vi "MGI Append String to Error Source.vi"(4 "Append to Warning? (F)":bool, 6 "Prepend? (F)":bool, 8 "Error In":errorcluster, 9 "String to Append":string) -> (0 "Error Out":errorcluster)   [LabVIEW 2016]
doc: "Append or Prepend the specified message to the input error source string if error exists.\n\nAuthored by Shawn Walpole\nsupport@mooregoodideas.com\nwww.mooregoodideas.com\n\nCopyright (c) 2010, Moore Good Ideas, Inc.\n\nAll rights reserved.\n\nRedistribution and use in source and binary forms, with or without modification, are permitted provided that the following conditions are met:\n\n * Redistributions of source code must retain the above copyright notice, this list of conditions and the following disclaimer.\n * Redistributions in binary form must reproduce the above copyright notice, this list of conditions and the following disclaimer in the documentation and/or other materials provided with the distribution.\n * Neither the name of Moore Good Ideas, Inc. nor the names of its contributors may be used to endorse or promote products derived from this software without specific prior written permission.\n\nTHIS SOFTWARE IS PROVIDED BY THE COPYRIGHT HOLDERS AND CONTRIBUTORS \"AS IS\" AND ANY EXPRESS OR IMPLIED WARRANTIES, INCLUDING, BUT NOT LIMITED TO, THE IMPLIED WARRANTIES OF MERCHANTABILITY AND FITNESS FOR A PARTICULAR PURPOSE ARE DISCLAIMED. IN NO EVENT SHALL THE COPYRIGHT OWNER OR CONTRIBUTORS BE LIABLE FOR ANY DIRECT, INDIRECT, INCIDENTAL, SPECIAL, EXEMPLARY, OR CONSEQUENTIAL DAMAGES (INCLUDING, BUT NOT LIMITED TO, PROCUREMENT OF SUBSTITUTE GOODS OR SERVICES; LOSS OF USE, DATA, OR PROFITS; OR BUSINESS INTERRUPTION) HOWEVER CAUSED AND ON ANY THEORY OF LIABILITY, WHETHER IN CONTRACT, STRICT LIABILITY, OR TORT (INCLUDING NEGLIGENCE OR OTHERWISE) ARISING IN ANY WAY OUT OF THE USE OF THIS SOFTWARE, EVEN IF ADVISED OF THE POSSIBILITY OF SUCH DAMAGE."
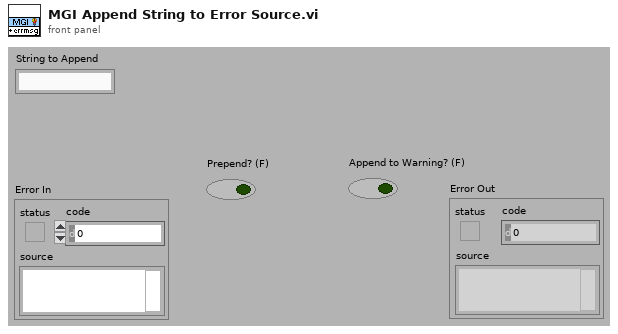
[diagram p1: front panel]
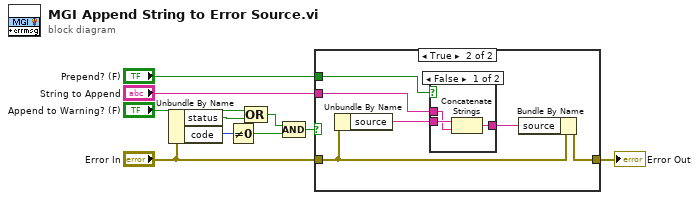
[diagram p0: block diagram]
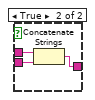
[diagram p3: hidden frame]
diagram:
  n1 = Unbundle By Name("Error In") -> ("status"=w10:bool, "code"=w7:i32)
  n2 = Not Equal To 0?(x=w7) -> (x != 0?=w6:bool)
  n3 = Compound Arithmetic op=OR("Append to Warning? (F)", w10) -> (w8:bool)
  n4 = Compound Arithmetic op=AND(w8, w6) -> (w5:bool)
  n5 = case shown="True" w5 {
    tunnel: "Error In" -> [w11 w17]
    tunnel: [w11 w16] -> w3
    tunnel: "Prepend? (F)" -> [_ w12]
    tunnel: "String to Append" -> [_ w13]
    frame False {
    }
    frame True {
      n6 = Unbundle By Name(w17) -> ("source"=w15:string)
      n7 = case shown="False" w12 {
        tunnel: w15 -> [w20 w23]
        tunnel: [w19 w21] -> w14
        tunnel: w13 -> [w18 w22]
        frame False {
          n8 = Concatenate Strings(w20, w18) -> (w19:string)
        }
        frame True {
          n9 = Concatenate Strings(w22, w23) -> (w21:string)
        }
      }
      n10 = Bundle By Name(cluster=w17, "source"=w14) -> (w16:errorcluster)
    }
  }
  "Error Out" <- w3
